vi "lstm-forward-pass-v1.vi"() -> ()   [LabVIEW 2020]
uses:
  <vilib>/Analysis/Matrix/Numeric/Conversions/Array To Matrix - RA.vi
  <vilib>/Analysis/Matrix/Numeric/Conversions/Matrix To Array - RM.vi
  <vilib>/Analysis/Matrix/NI_Matrix.lvlib
panel:
  out "Waveform Graph":dbl[][](graph)
  out "y true and predict":T1(graph)
  out "y predict values":dbl[](array[numeric])
  out "x waveform":dbl(graph)
  in  "cell 4 units":dbl
  in  "cell 3 units":dbl
  in  "cell 2 units":dbl
  out "t":dbl[][](array[numeric])
  in  "t data filepath":path
  out "y":dbl[][](array[numeric])
  in  "y data filepath":path
  out "X":dbl[][](array[numeric])
  in  "X data filepath":path
  in  "cell 1 units":dbl
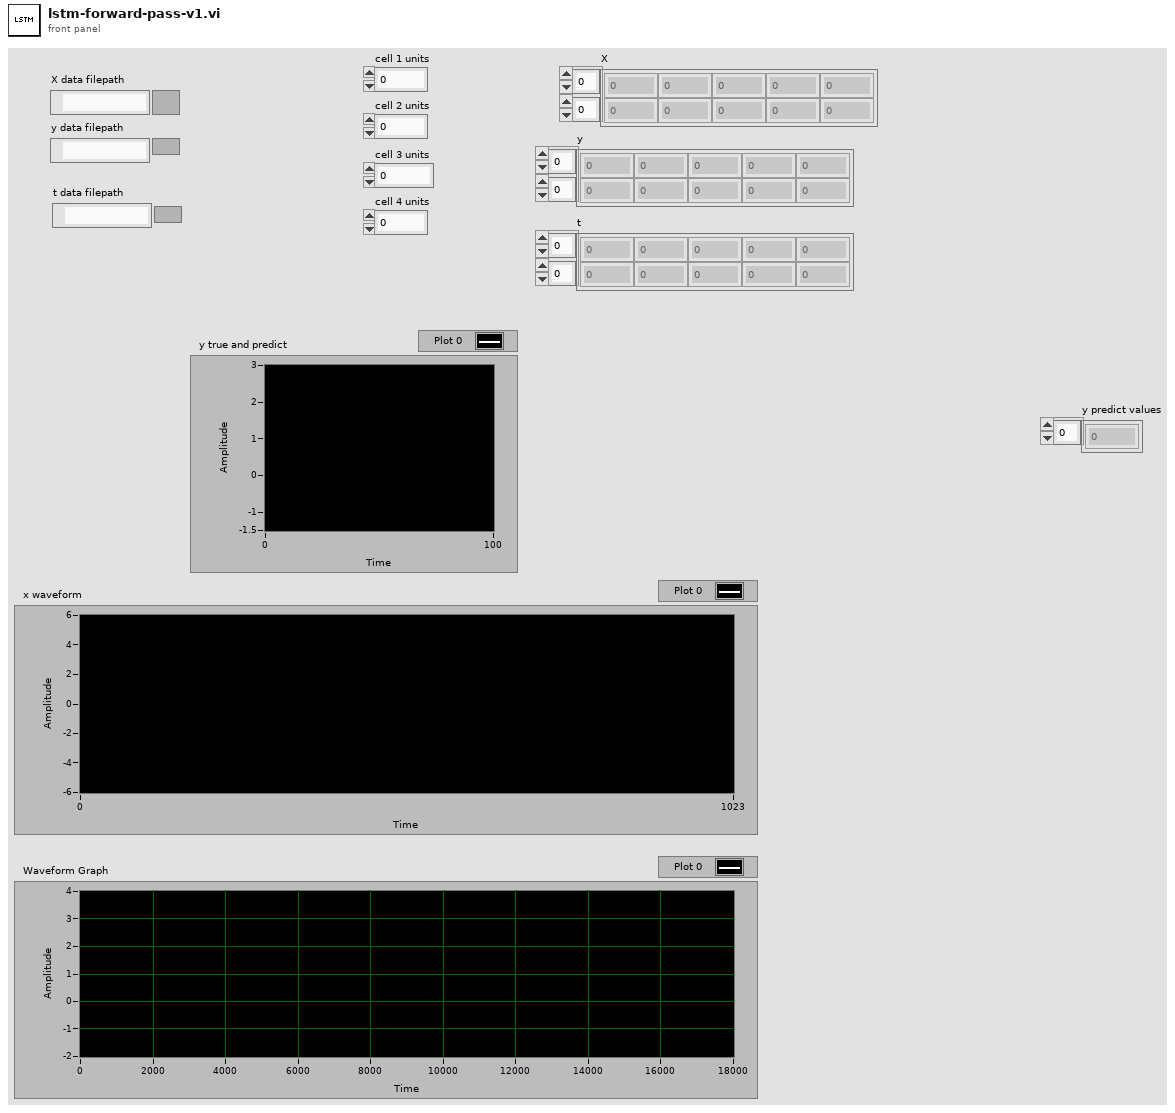
[diagram p1: front panel]
types:
  T1 = cluster{"Real Matrix Element":dbl, "Numeric":dbl}
  T2 = typedef "NI_Matrix.lvlib/RealMatrix.ctl" = dbl[][]
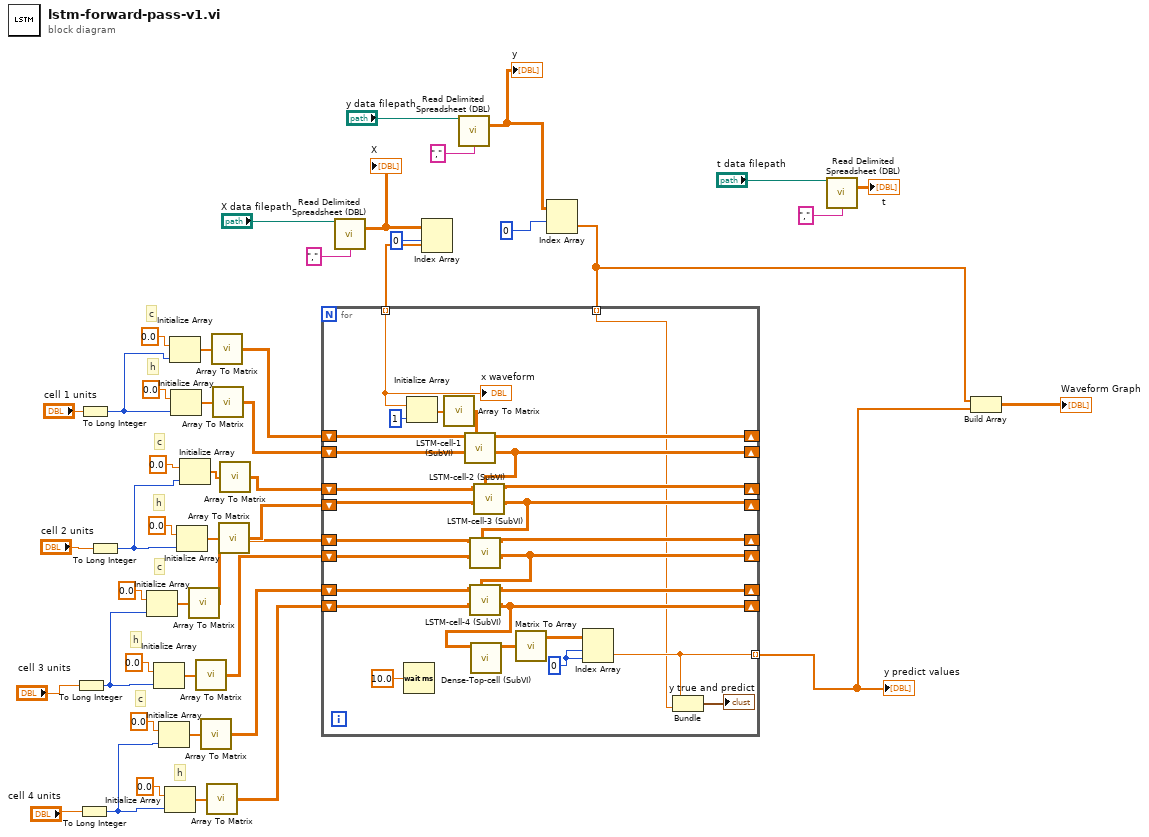
[diagram p0: block diagram]
diagram:
  # "c"
  # "c"
  # "c"
  # "c"
  # "h"
  # "h"
  # "h"
  # "h"
  n1 = To Long Integer(number="cell 3 units") -> (32bit integer=w17:i32)
  n2 = To Long Integer(number="cell 4 units") -> (32bit integer=w12:i32)
  n3 = To Long Integer(number="cell 1 units") -> (32bit integer=w24:i32)
  n4 = To Long Integer(number="cell 2 units") -> (32bit integer=w21:i32)
  n5 = Initialize Array(0.0, w17) -> (w18:dbl[])
  n6 = Initialize Array(0.0, w17) -> (w32:dbl[])
  n7 = Initialize Array(0.0, w12) -> (w13:dbl[])
  n8 = Initialize Array(0.0, w12) -> (w29:dbl[])
  n9 = Initialize Array(0.0, w24) -> (w25:dbl[])
  n10 = Initialize Array(0.0, w24) -> (w45:dbl[])
  n11 = Initialize Array(0.0, w21) -> (w35:dbl[])
  n12 = Initialize Array(0.0, w21) -> (w22:dbl[])
  n13 = call-poly <vilib>:"Array To Matrix.vi"("Real 1D Array"=w18) -> ("Real Matrix (Column Vector)"=w16:T2)
  n14 = call-poly <vilib>:"Array To Matrix.vi"("Real 1D Array"=w32) -> ("Real Matrix (Column Vector)"=w15:T2)
  n15 = call-poly <vilib>:"Array To Matrix.vi"("Real 1D Array"=w13) -> ("Real Matrix (Column Vector)"=w5:T2)
  n16 = call-poly <vilib>:"Array To Matrix.vi"("Real 1D Array"=w29) -> ("Real Matrix (Column Vector)"=w4:T2)
  n17 = call-poly <vilib>:"Array To Matrix.vi"("Real 1D Array"=w25) -> ("Real Matrix (Column Vector)"=w6:T2)
  n18 = call-poly <vilib>:"Array To Matrix.vi"("Real 1D Array"=w45) -> ("Real Matrix (Column Vector)"=w28:T2)
  n19 = call-poly <vilib>:"Array To Matrix.vi"("Real 1D Array"=w35) -> ("Real Matrix (Column Vector)"=w27:T2)
  n20 = call-poly <vilib>:"Array To Matrix.vi"("Real 1D Array"=w22) -> ("Real Matrix (Column Vector)"=w20:T2)
  n21 = call <vilib>:"Read Delimited Spreadsheet (DBL).vi"("file path (dialog if empty)"="X data filepath", "delimiter (\\t)"=",") -> ("all rows"=w11:dbl[][])  [unwired: 8 in, 5 out]
  "X" <- w11
  n22 = Index Array(array=w11, index (row)=0) -> (element=w9:dbl[])  [unwired: 1 in]
  n23 = call <vilib>:"Read Delimited Spreadsheet (DBL).vi"("file path (dialog if empty)"="y data filepath", "delimiter (\\t)"=",") -> ("all rows"=w7:dbl[][])  [unwired: 8 in, 5 out]
  "y" <- w7
  n24 = Index Array(array=w7, index (row)=0) -> (element=w3:dbl[])  [unwired: 1 in]
  n25 = for {
    shift-right: [w62] -> _
    shift-left: w28 -> [w74]
    shift-right: [w59] -> _
    shift-left: w27 -> [w61]
    shift-right: [w65] -> _
    shift-left: w6 -> [w73]
    shift-right: [w63] -> _
    shift-left: w20 -> [w64]
    shift-right: [w58] -> _
    shift-left: w16 -> [w60]
    shift-right: [w54] -> _
    shift-left: w15 -> [w57]
    shift-right: [w55] -> _
    shift-left: w5 -> [w56]
    shift-right: [w52] -> _
    shift-left: w4 -> [w53]
    tunnel: w9 -> [w69] mode=indexing
    tunnel: w3 -> [w50] mode=indexing
    tunnel: [w51] -> w2 mode=indexing
    w70 = 0
    n26 = Wait (ms)(milliseconds to wait=10.0) -> ()  [unwired: 1 out]
    n27 = Initialize Array(w69, 1) -> (w67:dbl[])
    n28 = call-poly <vilib>:"Array To Matrix.vi"("Real 1D Array"=w67) -> ("Real Matrix (Column Vector)"=w68:T2)
    n29 = call "LSTM-cell-1 (SubVI).vi"("x"=w68, "h"=w74, "c"=w73) -> ("h + 1"=w62:T2, "c + 1"=w65:T2)  [unwired: 7 in]
    n30 = call "LSTM-cell-2 (SubVI).vi"("x"=w62, "h"=w61, "c"=w64) -> ("h + 1"=w59:T2, "c + 1"=w63:T2)  [unwired: 7 in]
    n31 = call "LSTM-cell-3 (SubVI).vi"("x"=w59, "h"=w57, "c"=w60) -> ("h + 1"=w54:T2, "c + 1"=w58:T2)  [unwired: 7 in]
    n32 = call "LSTM-cell-4 (SubVI).vi"("x"=w54, "h"=w53, "c"=w56) -> ("h + 1"=w52:T2, "c + 1"=w55:T2)  [unwired: 7 in]
    n33 = call "Dense-Top-cell (SubVI).vi"("x_dense"=w52) -> ("y_out"=w66:T2)  [unwired: 10 in]
    n34 = call-poly <vilib>:"Matrix To Array.vi"("Real Matrix"=w66) -> ("Real 2D Array"=w71:dbl[][])
    n35 = Index Array(array=w71, index (row)=w70, index (col)=w70) -> (element=w51:dbl)
    n36 = Bundle("Real Matrix Element"=w51, "Numeric"=w50) -> (→"y true and predict":T1)  [unwired: 1 in]
    "x waveform" <- w69
  }
  "y predict values" <- w2
  n37 = call <vilib>:"Read Delimited Spreadsheet (DBL).vi"("file path (dialog if empty)"="t data filepath", "delimiter (\\t)"=",") -> ("all rows"=→"t":dbl[][])  [unwired: 8 in, 5 out]
  n38 = Build Array(w3, w2) -> (→"Waveform Graph":dbl[][])
